vi "sub_error_ignore.vi"(8 "error in":errorcluster caption="에러 입력(에러 없음)") -> (0 "error out":errorcluster caption="에러 출력")   [LabVIEW 2019]
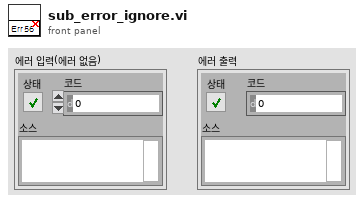
[diagram p1: front panel]
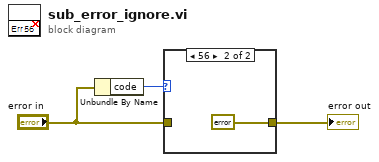
[diagram p0: block diagram]
diagram:
  n1 = Unbundle By Name("error in") -> ("code"=w1:i32)
  n2 = case shown="56" w1 {
    tunnel: "error in" -> [w4 _]
    tunnel: [w4 errorcluster {"status"=FALSE, "code"=0, "source"=""} ("error IO")] -> w3
    frame 0, Default {
    }
    frame 56 {
    }
  }
  "error out" <- w3
